vi "Write Value.vi"(8 "error in (no error)":errorcluster, 10 "Value":i32, 11 "Food in":refnum<class "Food.lvclass">) -> (0 "error out":errorcluster, 3 "Food out":refnum<class "Food.lvclass">)   [LabVIEW 2019, in "Food.lvclass"]
uses:
  Food.lvclass
  Food.lvclass/Food.ctl
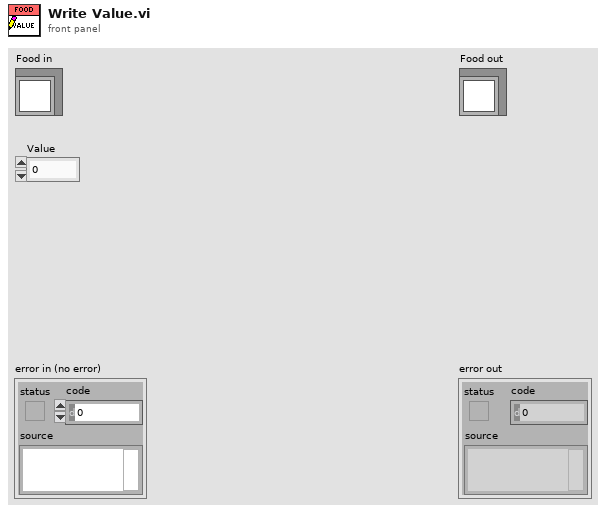
[diagram p1: front panel]
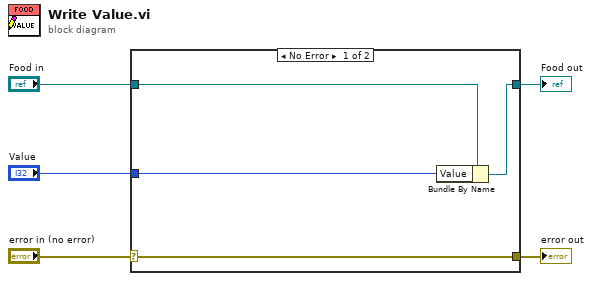
[diagram p0: block diagram]
diagram:
  n1 = case shown="No Error" "error in (no error)" {
    selector: "error in (no error)" -> [w9 w10]
    tunnel: [w9 w10] -> w4
    tunnel: [w7 w11] -> w2
    tunnel: "Food in" -> [w8 w11]
    tunnel: "Value" -> [w6 _]
    frame No Error {
      n2 = Bundle By Name(cluster=w8, "Value"=w6) -> (w7:refnum<class "Food.lvclass">)
    }
    frame Error {
    }
  }
  "error out" <- w4
  "Food out" <- w2
